vi "Subtract Polynomials (DBL).vi"(8 "threshold type":T1 items=["Absolute Value", "Relative Value"], 9 "threshold":dbl, 10 "Q(x)":dbl[](array[numeric]) format="%#.6g", 11 "P(x)":dbl[](array[numeric]) format="%#.6g") -> (0 "error":i32, 3 "P(x)-Q(x)":dbl[](array[numeric]) format="%#.6g")   [LabVIEW 2017, in "NI_AALPro.lvlib"]
doc: "Subtracts polynomial <B>Q(x)</B> from polynomial <B>P(x)</B>. The data types you wire to the <B>P(x)</B> and <B>Q(x)</B> inputs determine the polymorphic instance to use."
uses:
  <vilib>/Analysis/NI_AALPro.lvlib
  <vilib>/Analysis/polynomials.llb/Remove Zero Threshold Type.ctl
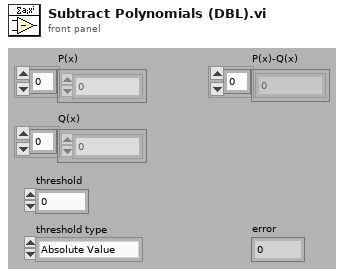
[diagram p1: front panel]
types:
  T1 = typedef "NI_AALPro.lvlib/Remove Zero Threshold Type.ctl" = u16
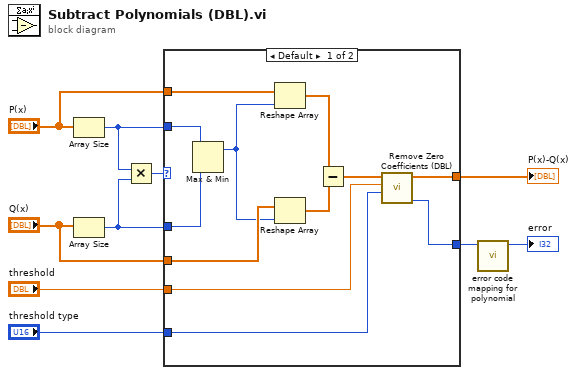
[diagram p0: block diagram]
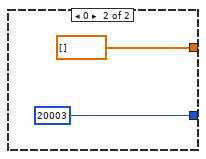
[diagram p2: hidden frame]
diagram:
  n1 = Array Size(array="P(x)") -> (size(s)=w6:i32)
  n2 = Array Size(array="Q(x)") -> (size(s)=w5:i32)
  n3 = Multiply(x=w6, y=w5) -> (x*y=w7:i32)
  n4 = case shown="Default" w7 {
    tunnel: w6 -> [w22 _]
    tunnel: w5 -> [w21 _]
    tunnel: "P(x)" -> [w16 _]
    tunnel: "Q(x)" -> [w17 _]
    tunnel: [w19 dbl[] []] -> w8
    tunnel: [w18 20003 ("empty array")] -> w4
    tunnel: "threshold" -> [w12 _]
    tunnel: "threshold type" -> [w11 _]
    frame Default {
      n5 = Max & Min(x=w22, y=w21) -> (max(x,y)=w15:i32)  [unwired: 1 out]
      n6 = Reshape Array(w16, w15) -> (w14:dbl[])
      n7 = Reshape Array(w17, w15) -> (w13:dbl[])
      n8 = Subtract(x=w14, y=w13) -> (x-y=w20:dbl[])
      n9 = call <vilib>:"Remove Zero Coefficients (DBL).vi"("threshold type"=w11, "threshold"=w12, "P(x) In"=w20) -> ("error"=w18:i32, "P(x) Out"=w19:dbl[])  [unwired: 6 in, 1 out]
    }
    frame 0 {
    }
  }
  "P(x)-Q(x)" <- w8
  n10 = call <vilib>:"error code mapping for polynomial.vi"("error in"=w4) -> ("error out"=→"error":i32)  [unwired: 10 in]
